vi "Get arrays without blanks.vi"(2 "String array in":string[](array[string]), 3 "Values in":dbl[](array[numeric]) format="%.6f", 7 "Booleans in":bool[](array[boolean])) -> (13 "Booleans out":bool[](array[boolean]), 16 "String array out":string[](array[string]), 17 "Values out":dbl[](array[numeric]) format="%.6f", 18 "Array size out":i32)   [LabVIEW 2020]
doc: "Returns the string array and related values and boolean arrays without white space string fields."
panel:
  out "Array size in":i32
  # "Returns the string array and related values and boolean arrays without white space string fields."
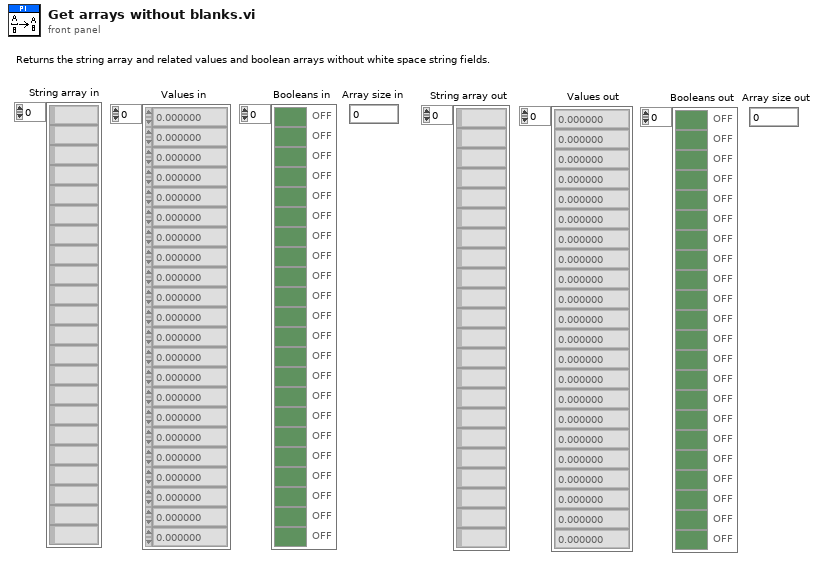
[diagram p1: front panel]
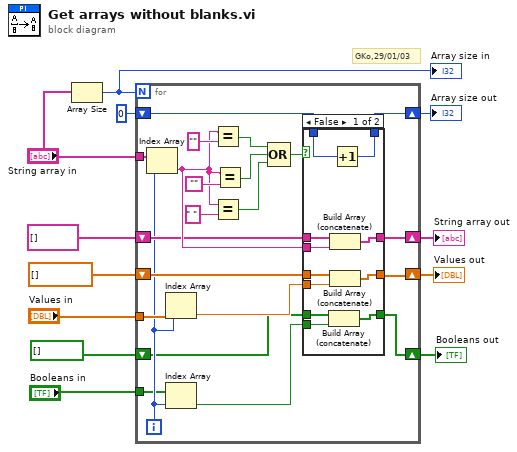
[diagram p0: block diagram]
diagram:
  # "GKo,29/01/03"
  n1 = Array Size(array="String array in") -> (size(s)=w10:i32)
  "Array size in" <- w10
  n2 = for {
    N: w10 -> [_]
    tunnel: "String array in" -> [w25]
    shift-right: [w26] -> w6
    shift-left: 0 -> [w27]
    shift-right: [w23] -> w5
    shift-left: string[] [] -> [w22]
    tunnel: "Values in" -> [w21]
    shift-right: [w20] -> w4
    shift-left: dbl[] [] -> [w19]
    tunnel: "Booleans in" -> [w16]
    shift-right: [w13] -> w1
    shift-left: bool[] [] ("Booleans in") -> [w15]
    i -> [w17]
    n3 = Index Array(array=w25, index=w17) -> (element=w24:string)
    n4 = Index Array(array=w21, index=w17) -> (element=w18:dbl)
    n5 = Index Array(array=w16, index=w17) -> (element=w14:bool)
    n6 = Equal?(x=w24, y="") -> (x = y?=w31:bool)
    n7 = Equal?(x=w24, y=" ") -> (x = y?=w29:bool)
    n8 = Equal?(x=w24, y="") -> (x = y?=w30:bool)
    n9 = Compound Arithmetic op=OR(w31, w30, w29) -> (w28:bool)
    n10 = case shown="False" w28 {
      tunnel: w27 -> [w45 w47]
      tunnel: [w38 w47] -> w26
      tunnel: w24 -> [w44 _]
      tunnel: [w43 w49] -> w23
      tunnel: w22 -> [w42 w49]
      tunnel: [w41 w48] -> w20
      tunnel: w19 -> [w40 w48]
      tunnel: w18 -> [w39 _]
      tunnel: w15 -> [w37 w46]
      tunnel: w14 -> [w36 _]
      tunnel: [w35 w46] -> w13
      frame False {
        n11 = Build Array (concatenate)(w37, w36) -> (w35:bool[])
        n12 = Build Array (concatenate)(w42, w44) -> (w43:string[])
        n13 = Build Array (concatenate)(w40, w39) -> (w41:dbl[])
        n14 = Increment(x=w45) -> (x+1=w38:i32)
      }
      frame True {
      }
    }
  }
  "String array out" <- w5
  "Values out" <- w4
  "Array size out" <- w6
  "Booleans out" <- w1
